vi "getGUID.vi"(8 "error in (no error)":errorcluster) -> (0 "error out":errorcluster, 3 "GUID":string)   [LabVIEW 2013, in "ProcessInfo.lvlib"]
uses:
  ProcessInfo.lvlib
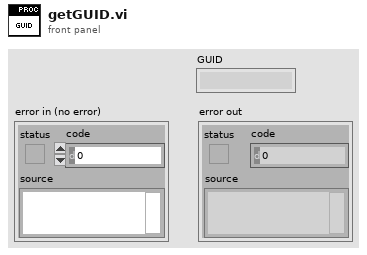
[diagram p1: front panel]
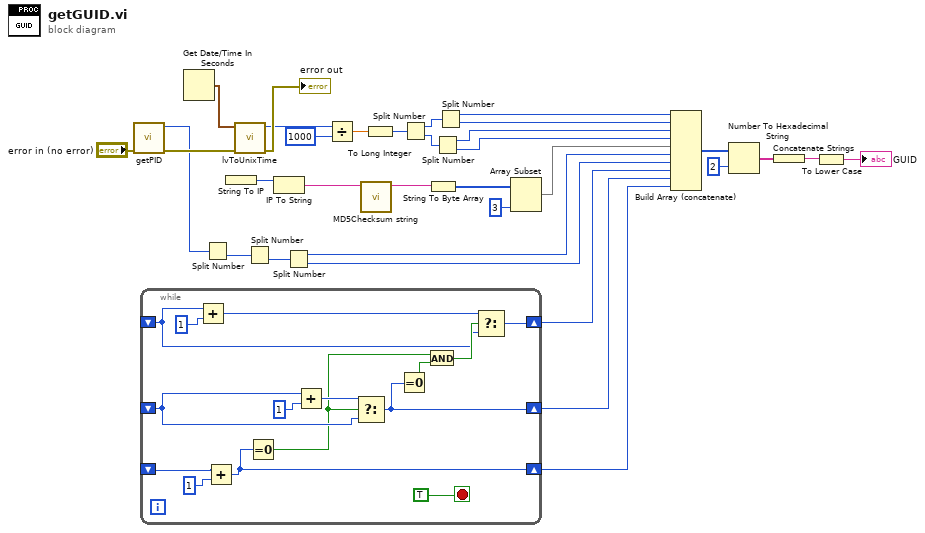
[diagram p0: block diagram]
diagram:
  n1 = call "getPID.vi"("error in (no error)"="error in (no error)") -> ("error out"=w4:errorcluster, "Current PID"=w3:i64)  [unwired: 9 in]
  n2 = while {
    shift-right: [w42] -> w26
    shift-left: _ -> [w47]
    shift-right: [w41] -> w25
    shift-left: _ -> [w43]
    shift-right: [w35] -> w24
    shift-left: _ -> [w34]
    stop <- TRUE stop-if-true
    n3 = Add(x=w34, y=u8 1) -> (x+y=w36:u8)
    n4 = Add(x=w47, y=u8 1) -> (x+y=w42:u8)
    n5 = Equal To 0?(x=w42) -> (x = 0?=w40:bool)
    n6 = Add(x=w43, y=u8 1) -> (x+y=w44:u8)
    n7 = Select(t=w44, s=w40, f=w43) -> (s? t:f=w41:u8)
    n8 = Equal To 0?(x=w41) -> (x = 0?=w39:bool)
    n9 = And(x=w40, y=w39) -> (x .and. y?=w37:bool)
    n10 = Select(t=w36, s=w37, f=w34) -> (s? t:f=w35:u8)
  }
  n11 = Get Date/Time In Seconds() -> (seconds since 1Jan1904=w6:timestamp)
  n12 = Split Number(x=w3) -> (lo(x)=w12:u32)  [unwired: 1 out]
  n13 = String To IP() -> (0:w5:u32)  [unwired: 1 in]
  n14 = call "lvToUnixTime.vi"("error in"=w4, "Local Time Stamp"=w6) -> ("error out"=→"error out":errorcluster, "Unix Time (in milliseconds)"=w7:u64)  [unwired: 8 in]
  n15 = Split Number(x=w12) -> (lo(x)=w13:u16)  [unwired: 1 out]
  n16 = IP To String(2:w5) -> (0:w32:string)  [unwired: 1 in]
  n17 = Split Number(x=w13) -> (hi(x)=w22:u8, lo(x)=w23:u8)
  n18 = Divide(x=w7, y=u64 1000) -> (x/y=w9:dbl)
  n19 = call <vilib>:"MD5Checksum string.vi"("Message String"=w32) -> ("MD5 message-digest"=w33:string)  [unwired: 10 in]
  n20 = To Long Integer(number=w9) -> (32bit integer=w14:i32)
  n21 = Split Number(x=w14) -> (hi(x)=w15:u16, lo(x)=w16:u16)
  n22 = String To Byte Array(string=w33) -> (unsigned byte array=w10:u8[])
  n23 = Split Number(x=w16) -> (hi(x)=w19:u8, lo(x)=w20:u8)
  n24 = Split Number(x=w15) -> (hi(x)=w17:u8, lo(x)=w18:u8)
  n25 = Array Subset(array=w10, length=3) -> (w21:u8[])  [unwired: 1 in]
  n26 = Build Array (concatenate)(w17, w18, w19, w20, w21, w22, w23, w24, w25, w26) -> (w28:u8[])
  n27 = Number To Hexadecimal String(1:i16 2 ("width (-)"), 2:w28) -> (0:w30:string[])
  n28 = Concatenate Strings(w30) -> (w31:string)
  n29 = To Lower Case(string=w31) -> (all lower case string=→"GUID":string)
